vi "Process Pretrigger Data.vi"(2 "Numeric 2":i32, 3 "Numeric 3":sgl, 4 "CH0 Raw Data":sgl[](array[numeric]), 5 "Array":sgl[][](array[numeric])) -> (0 "Boolean":bool, 1 "Numeric":i32)   [LabVIEW 2019]
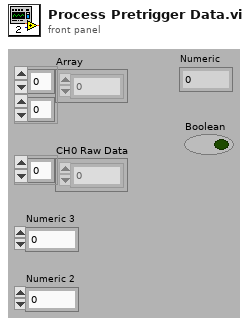
[diagram p1: front panel]
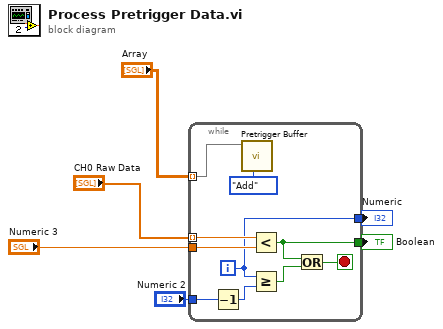
[diagram p0: block diagram]
diagram:
  n1 = while {
    tunnel: "Array" -> [w7] mode=indexing
    tunnel: "CH0 Raw Data" -> [w15] mode=indexing
    tunnel: "Numeric 3" -> [w14]
    tunnel: [w11] -> w4
    tunnel: "Numeric 2" -> [w9]
    tunnel: [w8] -> w5
    i -> [w8]
    stop <- w10 stop-if-true
    n2 = Decrement(x=w9) -> (x-1=w13:i32)
    n3 = call "Pretrigger Buffer.vi"("Mode"=enum16{"Initialize", "Add", "Read"}."Add", "New Data"=w7) -> ()  [unwired: 7 in, 2 out]
    n4 = Less?(x=w15, y=w14) -> (x < y?=w11:bool)
    n5 = Greater Or Equal?(x=w8, y=w13) -> (x >= y?=w12:bool)
    n6 = Or(x=w11, y=w12) -> (x .or. y?=w10:bool)
  }
  "Numeric" <- w5
  "Boolean" <- w4
